vi "NI VeriStand - Set Channel Values by Block Data Reference.vi"(8 "error in (no error)":errorcluster, 10 "Values Array in":dbl[](array[numeric]), 11 "Block Data Ref":T1[](array[typedef]) {"Data Reference" format="%.0x"}) -> (0 "error out":errorcluster, 2 "Values Array out":dbl[](array[numeric]), 3 "Block Data Ref dup":T1[](array[typedef]) {"Data Reference" format="%.0x"})   [LabVIEW 2020, in "Custom Device API.lvlib"]
doc: "Sets the values of the inline custom device channels specified by <B>Block Data Ref</B>. You can use this VI to get multiple channel values at one time. Use the Get Channel Block Data References VI to get the channel data references for this VI.\n\nYou can use this VI in the Execute Model case of an Inline Model Interface custom device, or in the Read Data from HW or Write Data to HW cases of an Inline Hardware Interface custom device. Do not use this VI outside of an inline custom device."
uses:
  <vilib>/NI VeriStand/Custom Device API/Custom Device API.lvlib
  <vilib>/NI VeriStand/Custom Device API/Block Data Reference.ctl
  <vilib>/NI VeriStand/Custom Device API/Data Reference.ctl
  <vilib>/NI VeriStand/Custom Device API/Global Data Refs.vi
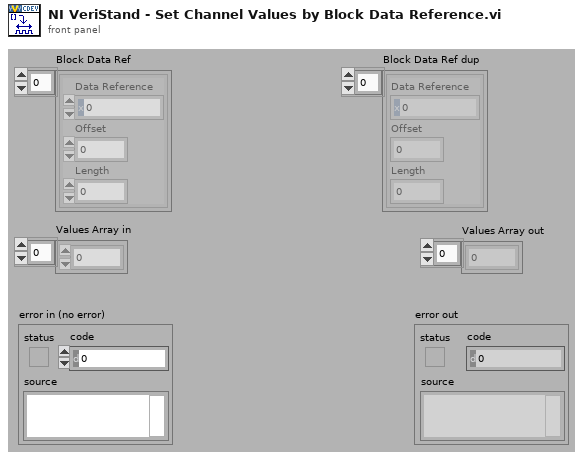
[diagram p1: front panel]
types:
  T1 = typedef "Custom Device API.lvlib/Block Data Reference.ctl" = cluster{"Data Reference":T2, "Offset":u64, "Length":u64}
  T2 = typedef "Custom Device API.lvlib/Data Reference.ctl" = i32
  T3 = typedef "Custom Device API.lvlib/Data Table Ref.ctl" = cluster{"Ptr.Beg":u64, "Ptr.End":u64}
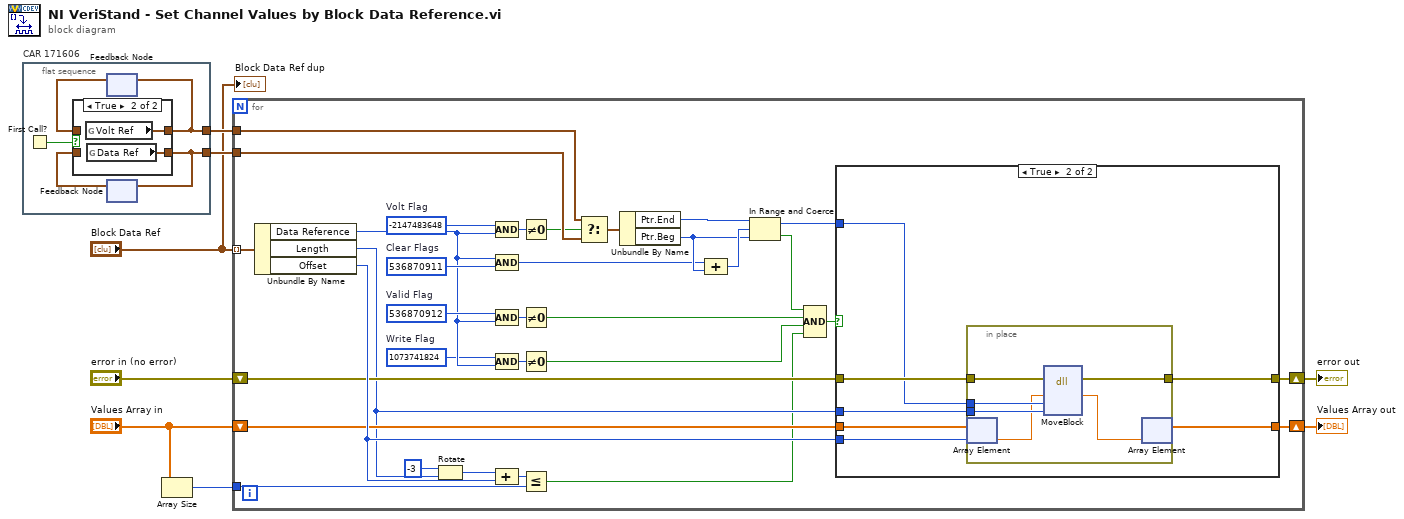
[diagram p0: block diagram]
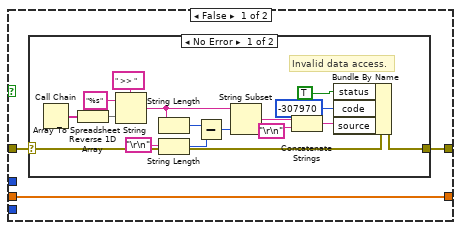
[diagram p3: hidden frame]
diagram:
  n1 = flat-sequence "CAR 171606" {
    tunnel: [w10] -> w3
    tunnel: [w9] -> w2
    frame #0 {
      n2 = First Call?() -> (First Call?: T/F=w13:bool)
      n3 = feedback #1() -> (w12:T3)  [unwired: 1 out]
      n4 = feedback #2() -> (w11:T3)  [unwired: 1 out]
      n5 = case shown="True" w13 {
        tunnel: [w15 w17] -> w10
        tunnel: w12 -> [w15 _]
        tunnel: [w14 w16] -> w9
        tunnel: w11 -> [w14 _]
        frame False {
        }
        frame True {
          n6 = global read "Global Data Refs.vi" "Volt Ref"() -> (w17:T3)
          n7 = global read "Global Data Refs.vi" "Data Ref"() -> (w16:T3)
        }
      }
      n8 = feedback-in #1(w10) -> ()
      n9 = feedback-in #2(w9) -> ()
    }
  }
  n10 = Array Size(array="Values Array in") -> (size(s)=w4:i32)
  n11 = for {
    tunnel: "Block Data Ref" -> [w33] mode=indexing
    shift-right: [w42] -> w8
    shift-left: "error in (no error)" -> [w43]
    tunnel: w3 -> [w30]
    tunnel: w2 -> [w49]
    shift-right: [w29] -> w6
    shift-left: "Values Array in" -> [w28]
    tunnel: w4 -> [w22]
    w18 = 1073741824  # Write Flag
    w35 = 536870912  # Valid Flag
    w37 = 536870911  # Clear Flags
    w40 = -2147483648  # Volt Flag
    n12 = Unbundle By Name(w33) -> ("Data Reference"=w26:T2, "Length"=w24:u64, "Offset"=w50:u64)
    n13 = Rotate(1:w24, 2:i8 -3 ("y")) -> (0:w20:u64)
    n14 = Compound Arithmetic op=AND(w40, w26) -> (w41:T2)
    n15 = Compound Arithmetic op=AND(w26, w37) -> (w31:T2)
    n16 = Compound Arithmetic op=AND(w35, w26) -> (w34:T2)
    n17 = Compound Arithmetic op=AND(w18, w26) -> (w27:T2)
    n18 = Compound Arithmetic op=ADD(w20, w50) -> (w23:u64)
    n19 = Not Equal To 0?(x=w41) -> (x != 0?=w39:bool)
    n20 = Not Equal To 0?(x=w34) -> (x != 0?=w32:bool)
    n21 = Not Equal To 0?(x=w27) -> (x != 0?=w25:bool)
    n22 = Less Or Equal?(x=w23, y=w22) -> (x <= y?=w21:bool)
    n23 = Select(t=w30, s=w39, f=w49) -> (s? t:f=w38:T3)
    n24 = Unbundle By Name(w38) -> ("Ptr.End"=w45:u64, "Ptr.Beg"=w44:u64)
    n25 = Compound Arithmetic op=ADD(w31, w44) -> (w48:u64)
    n26 = In Range and Coerce(upper limit=w45, x=w48, lower limit=w44) -> (coerced(x)=w47:u64, In Range?=w46:bool)
    n27 = Compound Arithmetic op=AND(w46, w32, w25, w21) -> (w36:bool)
    n28 = case shown="True" w36 {
      tunnel: w43 -> [w52 w77]
      tunnel: [w51 w76] -> w42
      tunnel: w47 -> [_ w74]
      tunnel: w24 -> [_ w75]
      tunnel: [w53 w72] -> w29
      tunnel: w28 -> [w53 w73]
      tunnel: w50 -> [_ w71]
      frame False {
        n29 = case shown="No Error" w52 {
          selector: w52 -> [w66 w70]
          tunnel: [w69 w70] -> w51
          frame No Error {
            # "Invalid data access."
            n30 = Call Chain() -> (call chain=w55:string[])
            n31 = Reverse 1D Array(array=w55) -> (reversed array=w62:string[])
            n32 = Array To Spreadsheet String(delimiter (Tab)=" >> ", array=w62, 3:"%s" ("format string")) -> (spreadsheet string=w63:string)
            n33 = String Length(string=w63) -> (length=w61:i32)
            n34 = String Length(string="\r\n") -> (length=w65:i32)
            n35 = Subtract(x=w61, y=w65) -> (x-y=w60:i32)
            n36 = String Subset(string=w63, length (rest)=w60) -> (substring=w56:string)  [unwired: 1 out]
            n37 = Concatenate Strings(w56, "\r\n") -> (w54:string)
            n38 = Bundle By Name(cluster=w66, "status"=TRUE, "code"=-307970, "source"=w54) -> (w69:errorcluster)
          }
          frame Error {
            # "Leave existing error."
          }
        }
      }
      frame True {
        n39 = in-place {
          in-place-border: w77 -> [w83]
          in-place-border: [w82] -> w76
          in-place-border: w75 -> [w81]
          in-place-border: w74 -> [w80]
          n40 = in-place-array #3(w73, w71) -> (w79:dbl)
          n41 = dll-call lib="LabVIEW" fn="MoveBlock"(error in=w83, "ps"=w79, "pd"=w80, "size"=w81) -> (error out=w82:errorcluster, "ps"=w78:dbl)  [unwired: 4 in, 2 out]
          n42 = in-place-array #3(w78) -> (w72:dbl[])  [unwired: 1 out]
        }
      }
    }
  }
  "Values Array out" <- w6
  "error out" <- w8
  "Block Data Ref dup" <- "Block Data Ref"
